vi "Update Logging Status.vi"(10 "Log File Trigger":bool, 11 "File Log Spec in":T1 {"File Node Ref" format="%.0x"}) -> (3 "File Log Spec out":T1 {"File Node Ref" format="%.0x"})   [LabVIEW 2027, in "Embedded Data Logger Engine.lvlib"]
uses:
  Embedded Data Logger Engine.lvlib
  File Logging Specification.ctl
  Group Logging Specification.ctl
  Group Buffer Data.ctl
  Property Specification.ctl
  <vilib>/NI VeriStand/Custom Device API/Custom Device Item Ref.ctl
  Shared/Segment Files By.ctl
  Logging State.ctl
  <vilib>/NI VeriStand/Custom Device API/Custom Device API.lvlib
  Shared/Embedded Data Logger Shared.lvlib
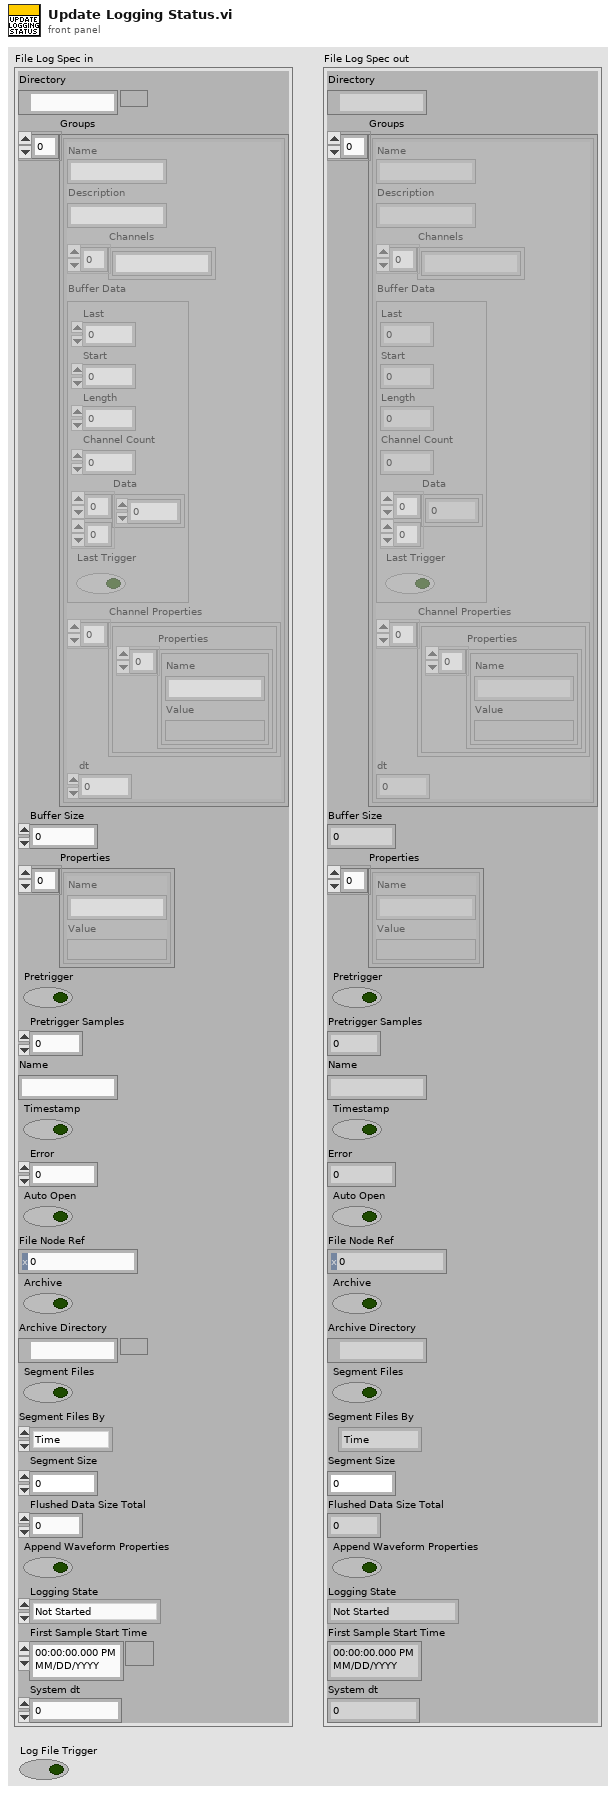
[diagram p1: front panel]
types:
  T1 = typedef "Embedded Data Logger Engine.lvlib/File Logging Specification.ctl" = cluster{"Directory":path, "Groups":T2[], "Buffer Size":i32, "Properties":T4[], "Pretrigger":bool, "Pretrigger Samples":i32, "Name":string, "Timestamp":bool, "Error":i32, "Auto Open":bool, "File Node Ref":T5, "Archive":bool, "Archive Directory":path, "Segment Files":bool, "Segment Files By":T6, "Segment Size":u32, "Flushed Data Size Total":u32, "Append Waveform Properties":bool, "Logging State":T7, "First Sample Start Time":timestamp, "System dt":dbl}
  T2 = typedef "Embedded Data Logger Engine.lvlib/Group Logging Specification.ctl" = cluster{"Name":string, "Description":string, "Channels":string[], "Buffer Data":T3, "Channel Properties":cluster{"Properties":T4[]}[], "dt":dbl}
  T3 = typedef "Embedded Data Logger Engine.lvlib/Group Buffer Data.ctl" = cluster{"Last":i32, "Start":i32, "Length":i32, "Channel Count":i32, "Data":dbl[][], "Last Trigger":bool}
  T4 = typedef "Embedded Data Logger Engine.lvlib/Property Specification.ctl" = cluster{"Name":string, "Value":variant}
  T5 = typedef "Custom Device API.lvlib/Custom Device Item Ref.ctl" = u64
  T6 = typedef "Embedded Data Logger Shared.lvlib/Segment Files By.ctl" = enum16{"Time", "Size"}
  T7 = typedef "Embedded Data Logger Engine.lvlib/Logging State.ctl" = enum16{"Not Started", "Continous Logging", "Paused", "Discontinous Logging"}
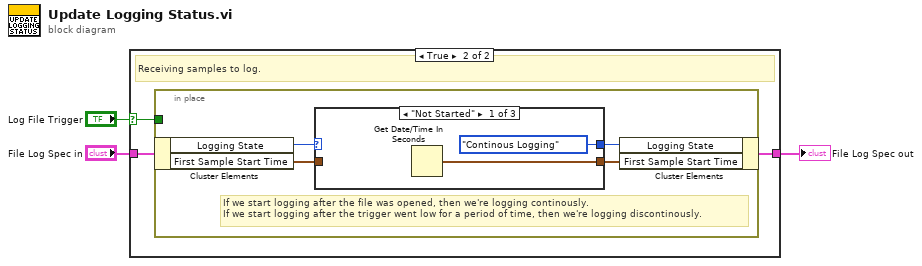
[diagram p0: block diagram]
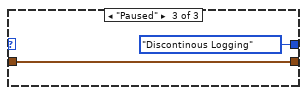
[diagram p4: hidden frame]
diagram:
  n1 = case shown="True" "Log File Trigger" {
    selector: "Log File Trigger" -> [_ w5]
    tunnel: "File Log Spec in" -> [w4 w7]
    tunnel: [w4 w6] -> w2
    frame False {
      # "Receiving pre-trigger samples."
    }
    frame True {
      # "Receiving samples to log."
      n2 = in-place {
        in-place-border: w5 -> [_]
        # "If we start logging after the file was opened, then we're logging continously.\nIf we start logging after the trigger went low for a period of time, then we're logging discontinously."
        n3 = in-place-cluster #1(w7) -> ("Logging State"=w11:T7, "First Sample Start Time"=w9:timestamp)
        n4 = case shown="\"Not Started\"" w11 {
          selector: w11 -> [_ w15 _]
          tunnel: [Logging_State."Continous Logging" ("Logging State") w15 Logging_State."Discontinous Logging" ("Logging State")] -> w10
          tunnel: w9 -> [_ w14 w16]
          tunnel: [w12 w14 w16] -> w8
          frame "Not Started" {
            n5 = Get Date/Time In Seconds() -> (seconds since 1Jan1904=w12:timestamp)
          }
          frame "Continous Logging", "Discontinous Logging" {
          }
          frame "Paused" {
          }
        }
        n6 = in-place-cluster #1("Logging State"=w10, "First Sample Start Time"=w8) -> (w6:T1)
      }
    }
  }
  "File Log Spec out" <- w2
